vi "Configure.vi"(8 "error in (no error)":errorcluster, 11 "Caraya Item in":refnum<class "Caraya Item.lvclass">) -> (0 "error out":errorcluster, 3 "Caraya Item out":refnum<class "Caraya Item.lvclass">)   [LabVIEW 2019, in "Caraya Library.lvlib" / "Caraya Item.lvclass"]
uses:
  Caraya Item.lvclass
  Caraya Item.lvclass/Caraya Item.ctl
panel:
  in  "Path":path
  in  "Cancel":bool
  in  "OK":bool
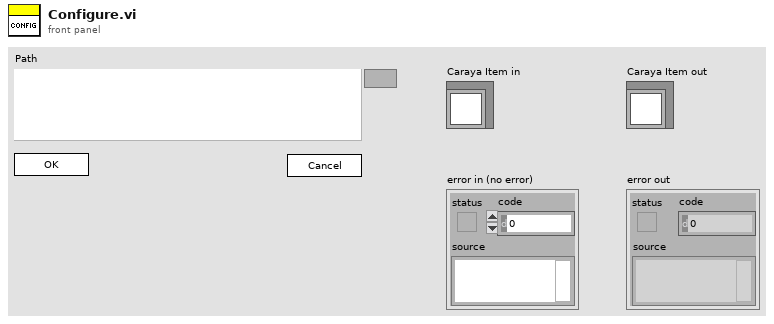
[diagram p1: front panel]
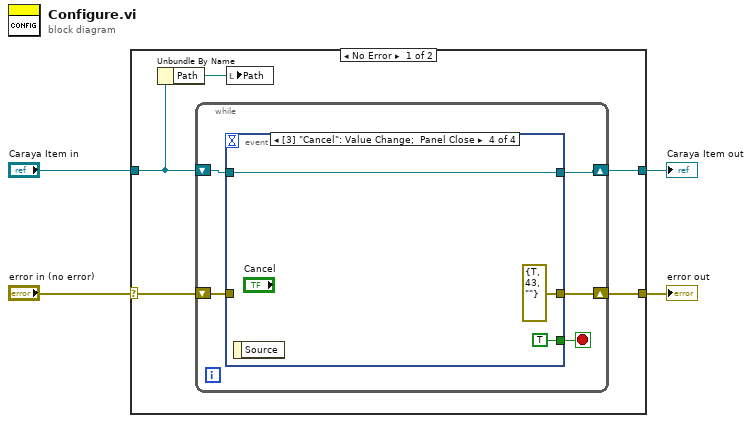
[diagram p0: block diagram]
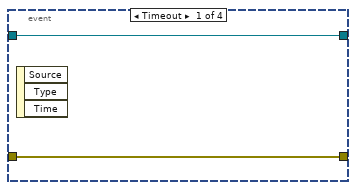
[diagram p2: hidden frame]
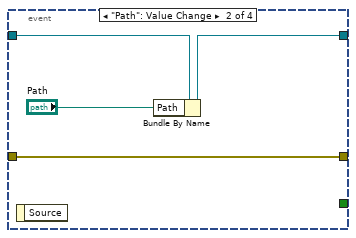
[diagram p3: hidden frame]
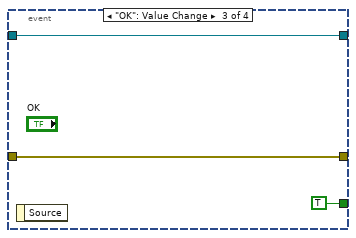
[diagram p4: hidden frame]
diagram:
  n1 = case shown="No Error" "error in (no error)" {
    selector: "error in (no error)" -> [w7 w28]
    tunnel: [w8 w28] -> w3
    tunnel: [w9 w27] -> w1
    tunnel: "Caraya Item in" -> [w6 w27]
    frame No Error {
      n2 = Unbundle By Name(w6) -> ("Path"=w5:path)
      n3 = while {
        shift-right: [w13] -> w8
        shift-left: w7 -> [w12]
        shift-right: [w14] -> w9
        shift-left: w6 -> [w11]
        stop <- w10 stop-if-true
        n4 = event shown="[3] \"Cancel\": Value Change;  Panel Close" {
          selector: _ -> [_ _ _ _]
          dyn-events: _ -> [_ _ _ _]
          timeout: _ -> [_ _ _ _]
          tunnel: [w16 w18 w23 w26] -> w14
          tunnel: w11 -> [w16 w20 w23 w26]
          tunnel: [w15 w19 w22 errorcluster {"status"=TRUE, "code"=43, "source"=""} ("error constant")] -> w13
          tunnel: w12 -> [w15 w19 w22 _]
          tunnel: [_ _ TRUE TRUE] -> w10
          event Timeout {
            n5 = event-data() -> ()  [unwired: 1 in, 3 out]
          }
          event "Path": Value Change {
            n6 = event-data() -> ()  [unwired: 1 in, 1 out]
            n7 = Bundle By Name(cluster=w20, "Path"="Path") -> (w18:refnum<class "Caraya Item.lvclass">)
          }
          event "OK": Value Change {
            n8 = event-data() -> ()  [unwired: 1 in, 1 out]
          }
          event "Cancel": Value Change; Panel Close {
            n9 = event-data() -> ()  [unwired: 1 in, 1 out]
          }
        }
      }
      n10 = local write "Path"(w5) -> ()
    }
    frame Error {
    }
  }
  "error out" <- w3
  "Caraya Item out" <- w1
